vi "Process.vi"(0 "reference in":refnum<class "TestView_Base.lvclass">, 5 "error in (no error)":errorcluster) -> (14 "reference out":refnum<class "TestView_Base.lvclass">, 19 "error out":errorcluster)   [LabVIEW 2017]
uses:
  TestView_Base.lvclass
  Components/MES_Base.lvlibp/Controls/Test.ctl
  Components/MES_Base.lvlibp/MES_Base.lvclass
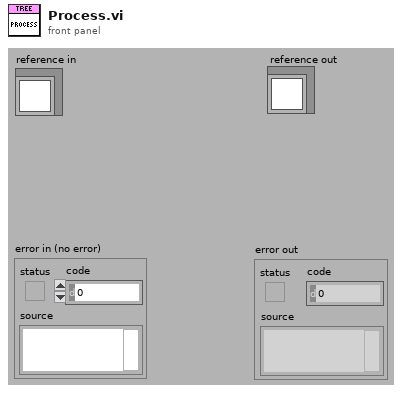
[diagram p1: front panel]
types:
  T1 = typedef "MES_Base.lvlibp/MES_Base.lvclass/Test.ctl" = cluster{"Code":string, "Name":string, "Description":string, "Group":string, "IsGroup":bool, "Tag":string, "Method":string, "Parrameter":string, "DataType":enum16{"NA", "String", "Boolean", "Int", "Dbl"}, "Value":variant, "Status":enum16{"Pending", "Pass", "Fail"}, "LimitLo":variant, "LimitHi":variant, "StringMatch":string, "BooleanMatch":bool, "DisplayFormat":string, "Units":string, "TestTime":dbl}
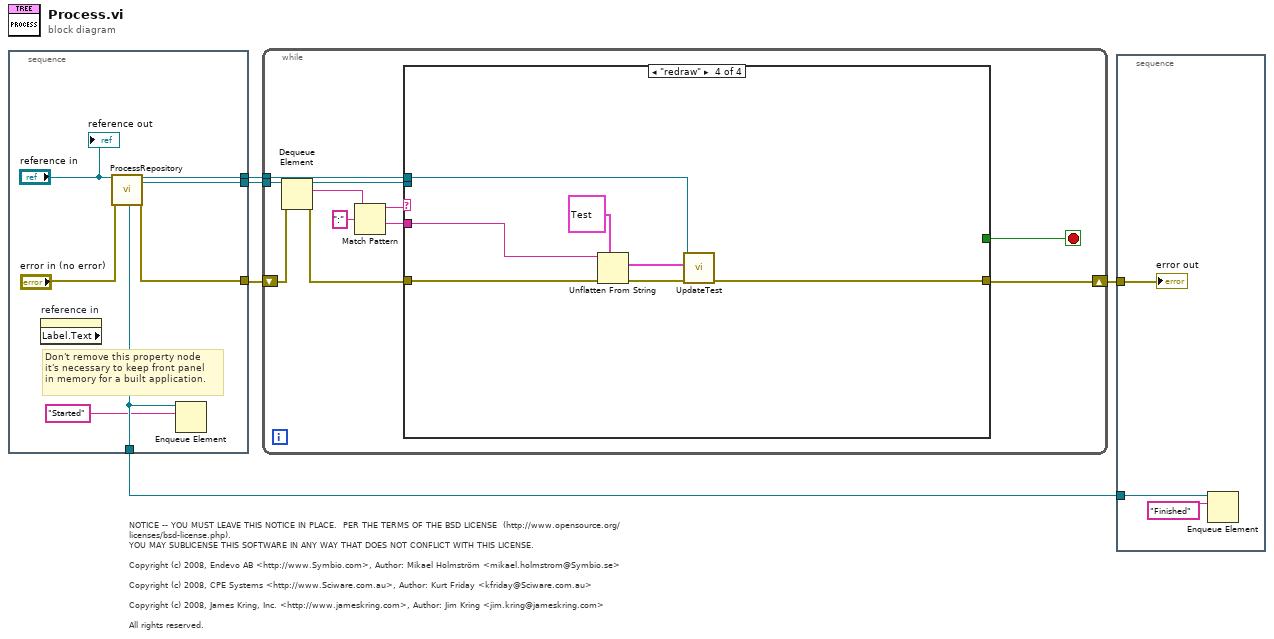
[diagram p0: block diagram]
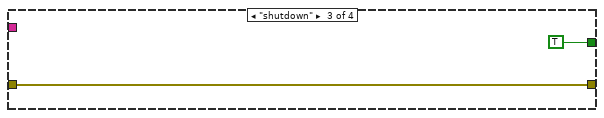
[diagram p4: hidden frame]
diagram:
  # "NOTICE -- YOU MUST LEAVE THIS NOTICE IN PLACE.  PER THE TERMS OF THE BSD LICENSE  (http://www.opensource.org/licenses/bsd-license.php).\nYOU MAY SUBLICENSE THIS SOFTWARE IN ANY WAY THAT DOES NOT CONFLICT WITH THIS LICENSE.\n\nCopyright (c) 2008, Endevo AB <http://www.Symbio.com>, Author: Mikael Holmström <mikael.holmstrom@Symbio.se>\n\nCopyright (c) 2008, CPE Systems <http://www.Sciware.com.au>, Author: Kurt Friday <kfriday@Sciware.com.au>\n\nCopyright (c) 2008, James Kring, Inc. <http://www.jameskring.com>, Author: Jim Kring <jim.kring@jameskring.com>\n\nAll rights reserved."
  n1 = stacked-sequence {
    tunnel: [w9] -> w5
    tunnel: [w12] -> w3
    tunnel: [w8] -> w2
    tunnel: [w7] -> w1
    frame #0 {
      # "Don't remove this property node\nit's necessary to keep front panel\nin memory for a built application."
      n2 = property on="reference in" class="LVClassControl (strict)" props=["Label", "Text"]() -> ()  [unwired: 2 in, 3 out]
      n3 = call "ProcessRepository.vi"("reference in"="reference in", "error in (no error)"="error in (no error)") -> ("ProcessSyncQueue"=w7:refnum<queue>, "reference out"=w12:refnum<class "TestView_Base.lvclass">, "ToProcessQueue"=w8:refnum<queue>, "error out"=w9:errorcluster)  [unwired: 11 in, 3 out]
      n4 = Enqueue Element(queue=w7, element="Started") -> ()  [unwired: 2 in, 3 out]
      "reference out" <- "reference in"
    }
  }
  n5 = while {
    shift-right: [w19] -> w4
    shift-left: w5 -> [w16]
    tunnel: w3 -> [w23]
    tunnel: w2 -> [w17]
    stop <- w13 stop-if-true
    n6 = Dequeue Element(queue=w17, error in (no error)=w16) -> (queue out=w18:refnum<queue>, element=w14:string, error out=w15:errorcluster)  [unwired: 1 in, 1 out]
    n7 = Match Pattern(string=w14, regular expression=":") -> (before substring=w21:string, after substring=w20:string)  [unwired: 1 in, 2 out]
    n8 = case shown="\"redraw\"" w21 {
      tunnel: w15 -> [w24 w25 w26 w33]
      tunnel: [w24 w25 w26 w32] -> w19
      tunnel: w18 -> [_ _ _ _]
      tunnel: w23 -> [_ _ _ w30]
      tunnel: w20 -> [_ _ _ w31]
      tunnel: [_ _ TRUE _] -> w13
      frame Default {
      }
      frame "Idle" {
      }
      frame "shutdown" {
      }
      frame "redraw" {
        n9 = Unflatten From String(type=T1 {"Code"="", "Name"="", "Description"="", "Group"="", "IsGroup"=FALSE, "Tag"="", "Method"="", "Parrameter"="", "DataType"=enum."String", "Value"=variant, "Status"=enum."Pass", "LimitLo"=variant, "LimitHi"=variant, "StringMatch"="", "BooleanMatch"=FALSE, "DisplayFormat"="", "Units"="", "TestTime"=0.0} ("Test"), binary string=w31, error in (no error)=w33) -> (value=w28:T1, error out=w34:errorcluster)  [unwired: 2 in, 1 out]
        n10 = call "UpdateTest.vi"("error in (no error)"=w34, "Test"=w28, "reference in"=w30) -> ("error out"=w32:errorcluster)  [unwired: 7 in, 1 out]
      }
    }
  }
  n11 = stacked-sequence {
    tunnel: w4 -> [w37]
    tunnel: w1 -> [w36]
    frame #0 {
      n12 = Enqueue Element(queue=w36, element="Finished") -> ()  [unwired: 2 in, 3 out]
      "error out" <- w37
    }
  }
